vi "sample7(BlockR All).vi"() -> ()   [LabVIEW 2020]
uses:
  <vilib>/Platform/TimedLoop/XDataNode/timing_clust.ctl
  <vilib>/Platform/TimedLoop/XDataNode/nitl_modes.ctl
  <vilib>/Platform/TimedLoop/XDataNode/wakeup.ctl
  <vilib>/Platform/TimedLoop/XDataNode/XDataNode.xnode
  <vilib>/Platform/TimedLoop/XDataNode/XDNodeRunTimeDep.lvlib
panel:
  out "CtrlTable":u8[][](array[numeric]) format="%02x"
  out "波形チャート":u32(graph)
  out "cycle time":u32
  out "ModelName":string
  out "err":errorcluster caption="エラー出力" {"code" format="%04x"}
  out "present load":i16
  in  "UPDATE":bool
  out "ACK":bool
  in  "TorqueEnable":bool
  in  "OffsetTime":u32=500
  in  "frequency":dbl=0.2 min=0.0 max=10.0 step=0.05
  in  "waveform":enum16{"sin", "square"}(ring)
  in  "Target ID":u8=1 max=253
  in  "Baudrate":u32=1000000 min=9600 max=3000000 step=100
  in  "COM":refnum<visa-resource-name> caption="COMポート"
  in  "wave":bool
  out "Chart":T1(graph)
  out "STOP2":bool
  out "present position":i32
  in  "STOP":bool
  in  "goal position":i32(knob) scale=262144.0..-262144.0
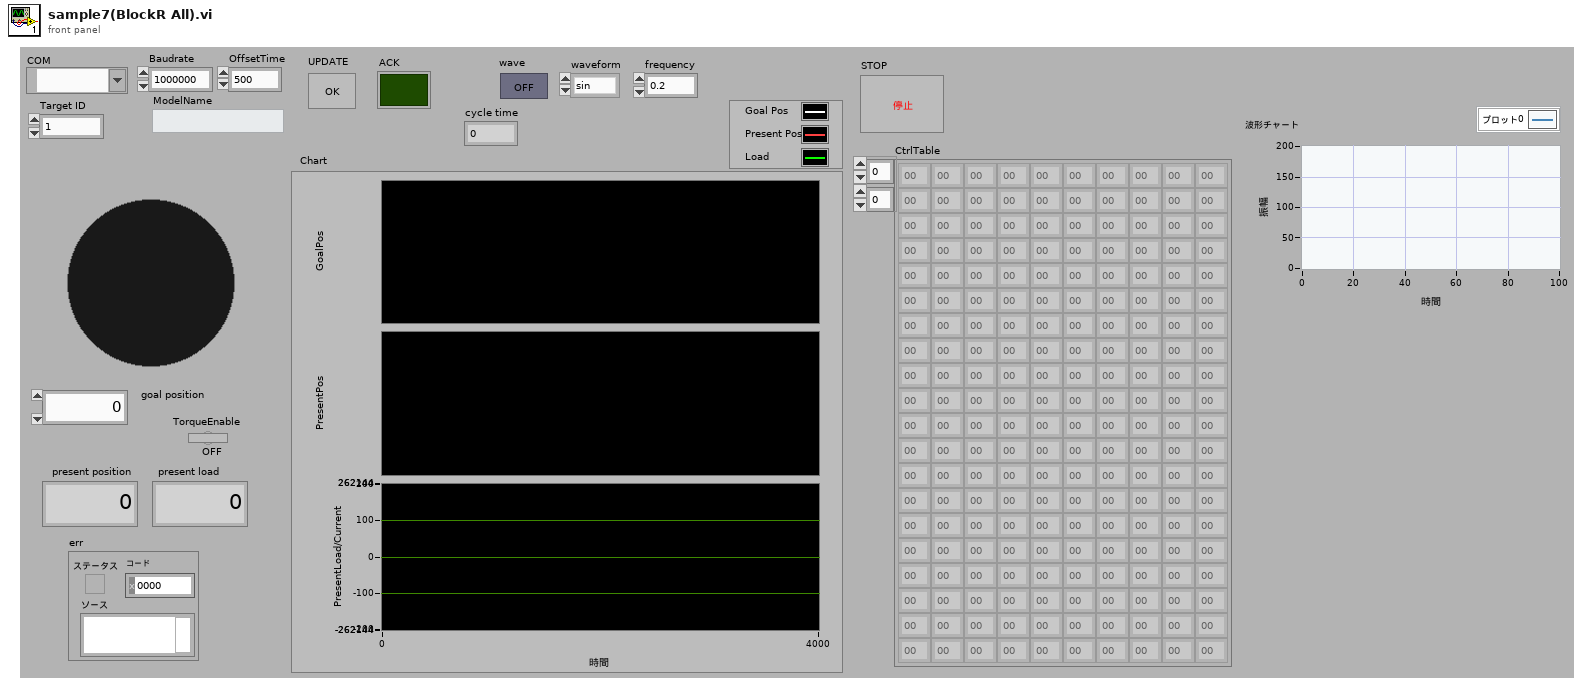
[diagram p1: front panel]
types:
  T1 = cluster{"goal position":i32, "present position":i32, "present load":i16}
  T2 = typedef "XDNodeRunTimeDep.lvlib/timing_clust.ctl" = cluster{"Expected End [f-1]":u64, "Actual End [f-1]":u64, "Finished Late? [f-1]":bool, "Expected End [i-1]":u64, "Actual End [i-1]":u64, "Finished Late? [i-1]":bool, "Expected Start [i]":u64, "Actual Start [i]":u64, "Expected Start [f]":u64, "Actual Start [f]":u64, "Source Name":string, "Structure Name":string, "Period":i64, "Deadline":i64, "Offset":i64, "Start":i64, "Priority":i32, "Timeout":i32, "Mode":T3, "Wakeup Reason":T4, "Error":errorcluster, "Source Type":string, "Secondary Source Type":string, "Global End Time":u64, "Global Start Time":u64, "Frame Duration":u64, "Iteration Duration":u64, "Assigned CPU":i32, "I/O Scan Engine Mode":u32}
  T3 = typedef "XDNodeRunTimeDep.lvlib/nitl_modes.ctl" = enum32{"No Change", "Process missed periods, maintain original phase", "Discard missed periods, maintain original phase", "Process missed periods, ignore original phase", "Discard missed periods, ignore original phase"}
  T4 = typedef "XDNodeRunTimeDep.lvlib/wakeup.ctl" = enum32{"Normal", "Aborted", "Asynchronous wakeup", "Timing source error", "Timed loop error", "Timeout"}
  T5 = cluster{"modelno":u16, "ModelName":string, "Type":enum8{"NONE", "DX", "AX", "RX", "EX", "MX", "XL320", "PRO", "PROP", "X", "Y"}, "MaxPosition":i32, "MinPosition":i32, "MaxAngle":dbl, "MinAngle":dbl, "MaxVelocity":i32, "MinVelocity":i32, "MaxPWM":i32, "MinPWM":i32, "VelocityRatio":dbl, "CurrentRatio":dbl, "PWMRatio":dbl}
  T6 = cluster{"ACK":bool, "ID":u8, "MaxPositionLimit":cluster{"address":u16, "width":u8, "limit":cluster{"max":i32, "min":i32}}, "MinPositionLimit":cluster{"address":u16, "width":u8, "limit":cluster{"max":i32, "min":i32}}, "TorqueEnable":cluster{"address":u16, "width":u8, "limit":cluster{"max":i32, "min":i32}}, "GoalPosition":cluster{"address":u16, "width":u8, "limit":cluster{"max":i32, "min":i32}}, "GoalVelocity":cluster{"address":u16, "width":u8, "limit":cluster{"max":i32, "min":i32}}, "PresentPosition":cluster{"address":u16, "width":u8, "limit":cluster{"max":i32, "min":i32}}, "PresentVelocity":cluster{"address":u16, "width":u8, "limit":cluster{"max":i32, "min":i32}}, "HardwareError":cluster{"address":u16, "width":u8, "limit":cluster{"max":i32, "min":i32}}}
  T7 = enum8{"NONE", "DX", "AX", "RX", "EX", "MX", "XL320", "PRO", "PROP", "X", "Y"}
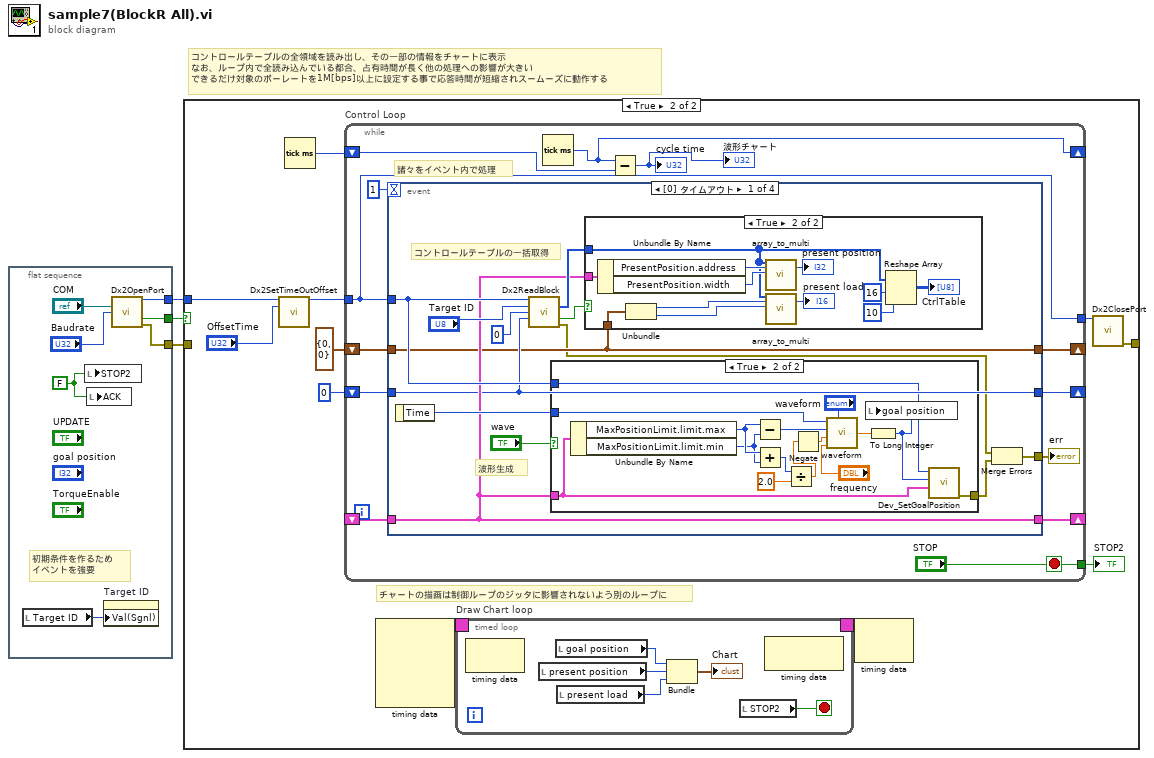
[diagram p0: block diagram]
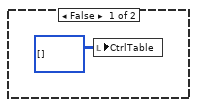
[diagram p4: hidden frame]
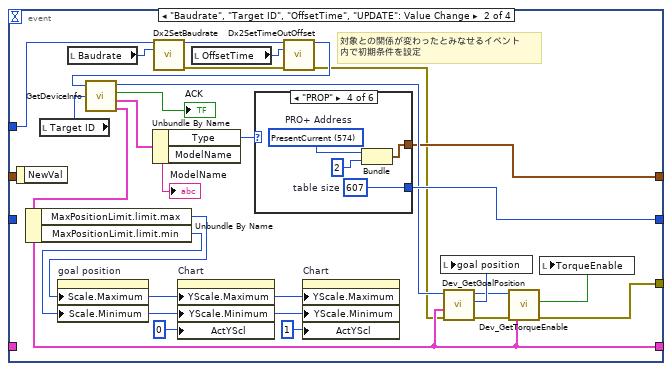
[diagram p5: hidden frame]
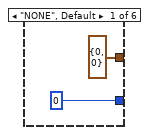
[diagram p6: hidden frame]
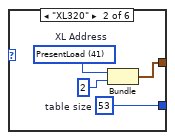
[diagram p7: hidden frame]
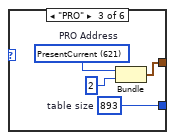
[diagram p8: hidden frame]
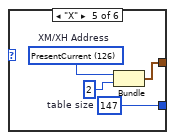
[diagram p9: hidden frame]
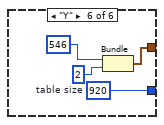
[diagram p10: hidden frame]
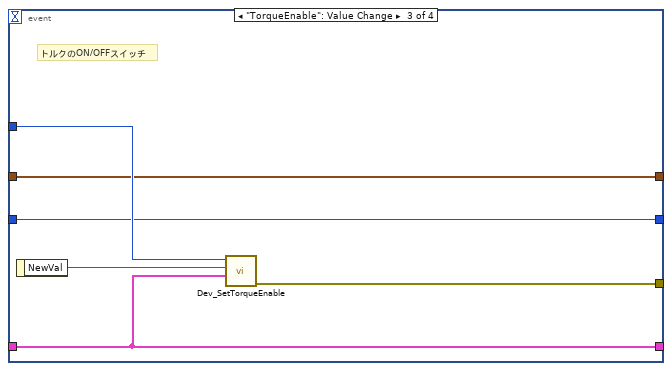
[diagram p11: hidden frame]
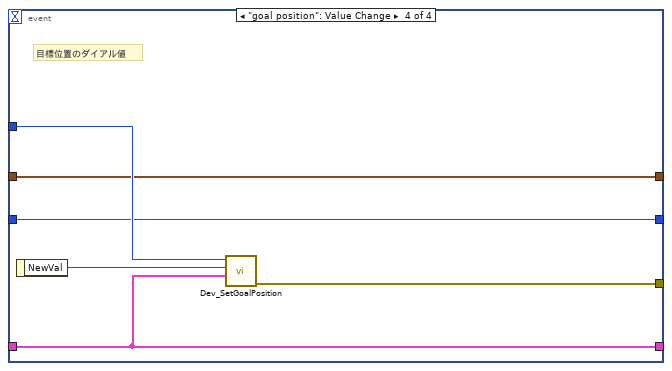
[diagram p12: hidden frame]
diagram:
  # "コントロールテーブルの全領域を読み出し、その一部の情報をチャートに表示\nなお、ループ内で全読み込んでいる都合、占有時間が長く他の処理への影響が大きい\nできるだけ対象のボーレートを1M[bps]以上に設定する事で応答時間が短縮されスームーズに動作する"
  n1 = flat-sequence {
    tunnel: [w10] -> w3
    tunnel: [w9] -> w2
    tunnel: [w8] -> w1
    frame #0 {
      w5 = FALSE ("停止 3")
      # "初期条件を作るため\nイベントを強要"
      n2 = local read "Target ID"() -> (w4:u8)
      n3 = local write "STOP2"(w5) -> ()
      n4 = local write "ACK"(w5) -> ()
      n5 = property on="Target ID" class="DigNum (指定)"("Val(Sgnl)"=w4) -> ()  [unwired: 2 in, 2 out]
      n6 = call "Dx2OpenPort.vi"("port"="COM", "baudrate"="Baudrate") -> ("dvid"=w9:u32, "成功"=w8:bool, "エラー出力"=w10:errorcluster)  [unwired: 11 in]
    }
  }
  n7 = case shown="TRUE" w1 {
    tunnel: w3 -> [w11 _]
    tunnel: w2 -> [_ w18]
    tunnel: [w11 w20] -> _
    frame False {
    }
    frame True {
      # "チャートの描画は制御ループのジッタに影響されないよう別のループに"
      n8 = call "Dx2SetTimeOutOffset.vi"("dvid in"=w18, "OffsetTime"="OffsetTime") -> ("dvid out"=w16:u32)  [unwired: 12 in, 1 out]
      n9 = Tick Count (ms)() -> (millisecond timer value=w12:u32)
      n10 = while "Control Loop" {
        shift-right: [w35] -> _
        shift-left: _ -> [w34]
        shift-right: [w33] -> _
        shift-left: u32 0 ("size") -> [w32]
        tunnel: w16 -> [w29]
        tunnel: ["STOP"] -> w17
        tunnel: [w29] -> w15
        shift-right: [w28] -> _
        shift-left: cluster{"XM/XM Address":u16, u8} {"XM/XM Address"=0, 0} -> [w27]
        shift-right: [w24] -> _
        shift-left: w12 -> [w25]
        stop <- "STOP" stop-if-true
        # "諸々をイベント内で処理"
        n11 = event shown="[0] タイムアウト" {
          selector: _ -> [_ _ _ _]
          dyn-events: _ -> [_ _ _ _]
          timeout: 1 -> [_ _ _ _]
          tunnel: [w41 w86 w127 w133] -> w35
          tunnel: w34 -> [w41 _ w127 w133]
          tunnel: [w38 w79 w124 w130] -> w26
          tunnel: [w40 w92 w126 w132] -> w33
          tunnel: w29 -> [w43 w91 w129 w134]
          tunnel: w32 -> [w40 _ w126 w132]
          tunnel: [w39 w87 w125 w131] -> w28
          tunnel: w27 -> [w39 _ w125 w131]
          event Timeout {
            # "波形生成"
            # "コントロールテーブルの一括取得"
            n12 = event-data() -> ("Time"=w44:u32)  [unwired: 1 in]
            n13 = call "Dx2ReadBlock.vi"("dvid in"=w43, "id"="Target ID", "address"=u16 0, "size"=w40) -> ("data out"=w47:u8[], "成功"=w46:bool, "エラー出力"=w36:errorcluster)  [unwired: 8 in, 1 out]
            n14 = case shown="TRUE" "wave" {
              tunnel: w41 -> [_ w51]
              tunnel: w44 -> [_ w63]
              tunnel: w43 -> [_ w61]
              tunnel: [_ w60] -> w37
              frame False {
              }
              frame True {
                n15 = Unbundle By Name(w51) -> ("MaxPositionLimit.limit.max"=w50:i32, "MaxPositionLimit.limit.min"=w49:i32)
                n16 = Subtract(x=w50, y=w49) -> (x-y=w57:i32)
                n17 = Add(x=w50, y=w49) -> (x+y=w56:i32)
                n18 = Divide(x=w56, y=2.0) -> (x/y=w55:dbl)
                n19 = Negate(x=w55) -> (-x=w52:dbl)
                n20 = call "waveform.vi"("time(ms)"=w63, "amplitude"=w57, "offset"=w52, "frequency"="frequency", "waveform"="waveform") -> ("wave"=w62:dbl)
                n21 = To Long Integer(number=w62) -> (32bit integer=w53:i32)
                n22 = local write "goal position"(w53) -> ()
                n23 = call "Dev_SetGoalPosition.vi"("ItemInfo"=w51, "goal position"=w53, "dvid in"=w61) -> ("エラー出力"=w60:errorcluster)  [unwired: 2 in, 2 out]
              }
            }
            n24 = case shown="TRUE" w46 {
              tunnel: w47 -> [_ w68]
              tunnel: w41 -> [_ w73]
              tunnel: w39 -> [_ w69]
              frame False {
                n25 = local write "CtrlTable"(u8[][] [] ("CtrlTable")) -> ()
              }
              frame True {
                n26 = Unbundle By Name(w73) -> ("PresentPosition.address"=w76:u16, "PresentPosition.width"=w75:u8)
                n27 = Unbundle(w69) -> ("XM/XM Address"=w71:u16, w70:u8)
                n28 = call "array_to_multi.vi"("array"=w68, "OffsetAddr"=w76, "length"=w75) -> ("uint32"=→"present position":u32)  [unwired: 16 in]
                n29 = call "array_to_multi.vi"("array"=w68, "OffsetAddr"=w71, "length"=w70) -> ("uint32"=→"present load":u32)  [unwired: 16 in]
                n30 = Reshape Array(w68, 16 ("次元サイズ"), 10 ("次元サイズ")) -> (→"CtrlTable":u8[][])
              }
            }
            n31 = Merge Errors(w36, w37) -> (w38:errorcluster)
          }
          event "Baudrate", "Target ID", "OffsetTime", "UPDATE": Value Change {
            # "対象との関係が変わったとみなせるイベント\n内で初期条件を設定"
            n32 = event-data() -> ()  [unwired: 1 in, 1 out]
            n33 = local read "Target ID"() -> (w95:u8)
            n34 = local read "Baudrate"() -> (w100:u32)
            n35 = call "Dx2SetBaudrate.vi"("dvid in"=w91, "Baudrate"=w100) -> ("dvid out"=w98:u32, "エラー出力"=w97:errorcluster)  [unwired: 11 in, 1 out]
            n36 = local read "OffsetTime"() -> (w99:u32)
            n37 = call "Dx2SetTimeOutOffset.vi"("dvid in"=w98, "OffsetTime"=w99, "エラー入力"=w97) -> ("dvid out"=w96:u32, "エラー出力"=w81:errorcluster)  [unwired: 11 in]
            n38 = call "GetDeviceInfo.vi"("dvid in"=w96, "Target ID"=w95) -> ("dvid out"=w90:u32, "matched"=→"ACK":bool, "ModelInfo"=w94:T5, "ItemInfo"=w86:T6)  [unwired: 1 in]
            n39 = Unbundle By Name(w86) -> ("MaxPositionLimit.limit.max"=w82:i32, "MaxPositionLimit.limit.min"=w83:i32)
            n40 = property on="goal position" class="Knob (指定)"("Scale.Maximum"=w82, "Scale.Minimum"=w83) -> ()  [unwired: 2 in, 2 out]
            n41 = Unbundle By Name(w94) -> ("Type"=w93:T7, "ModelName"=→"ModelName":string)
            n42 = property on="Chart" class="WFChart (指定)"("YScale.Maximum"=w82, "YScale.Minimum"=w83, "ActYScl"=0 ("アクティブYスケール")) -> ()  [unwired: 2 in, 2 out]
            n43 = case shown="\"PROP\"" w93 {
              tunnel: [u32 0 ("size") w107 w111 w115 w119 w123] -> w92
              tunnel: [cluster{"XM/XM Address":u16, u8} {"XM/XM Address"=0, 0} w104 w108 w113 w116 w121] -> w87
              frame "NONE", Default {
              }
              frame "XL320" {
                w106 = u16 41 items=["ModelNo"=0, "VersionOfFirmware"=2, "ID"=3, "Baudrate"=4, "ReturnDelayTime"=5, "CWAngleLimit"=6, "CCWAngleLimit"=8, "ControlMode"=11, "LimitTemperature"=12, "LowestLimitVoltage"=13, "HighestLimitVoltage"=14, "MaxTorque"=15, "StatusReturnLevel"=17, "AlarmShutdown"=18, "TorqueEnable"=24, "LED"=25, "DGain"=26, "IGain"=27, "PGain"=28, "GoalPosition"=30, "GoalVelocity"=32, "GoalTorque"=35, "PresentPosition"=37, "PresentSPeed"=39, "PresentLoad"=41, "PresentVoltage"=45, "PresentTemperature"=46, "RegistedInstruction"=47, "Moving"=49, "HardwareErrorStatus"=50, "Punch"=51]  # XL Address
                w107 = u32 53  # table size
                n44 = Bundle("XL Address"=w106, u8 2) -> (w104:cluster{"XL Address":u16, u8})  [unwired: 1 in]
              }
              frame "PRO" {
                w109 = u16 621 items=["ModelNo"=0, "ModelInfo"=2, "VersionOfFirmware"=6, "ID"=7, "Baudrate"=8, "ReturnDelayTime"=9, "OperationMode"=11, "HormingOffset"=13, "MovingThreshold"=17, "TemperatureLimit"=21, "MaxVoltageLimit"=22, "MinVoltageLimit"=24, "AccelerationLimit"=26, "TorqueLimit"=30, "VoltageLimit"=32, "MaxPositionLimit"=36, "MinPositionLimit"=40, "ExternalPortMode1"=44, "ExternalPortMode2"=45, "ExternalPortMode3"=46, "ExternalPortMode4"=47, "Shutdown"=48, "TorqueEnable"=562, "LED_Red"=563, "LED_Green"=564, "LED_Blue"=565, "VelocityIGain"=586, "VelocityPGain"=588, "PositionPGain"=594, "GoalPosition"=596, "GoalVelocity"=600, "GoalTorque"=604, "GoalAcceleration"=606, "Moving"=610, "PresentPosition"=611, "PresentVelocity"=615, "PresentCurrent"=621, "PresentInputVoltage"=623, "PresentTemperature"=625, "ExternalPortData1"=626, "ExternalPortData2"=628, "ExternalPortData3"=630, "ExternalPortData4"=632, "RegistedInstruction"=890, "StatusReturnLevel"=891, "HardwareError"=892]  # PRO Address
                w111 = u32 893  # table size
                n45 = Bundle("PRO Address"=w109, u8 2) -> (w108:cluster{"PRO Address":u16, u8})  [unwired: 1 in]
              }
              frame "PROP" {
                w112 = u16 574 items=["ModelNo"=0, "ModelInfo"=2, "VersionOfFirmware"=6, "ID"=7, "Baudrate"=8, "ReturnDelayTime"=9, "DriveMode"=10, "OperationMode"=11, "HormingOffset"=20, "MovingThreshold"=24, "TemperatureLimit"=31, "MaxVoltageLimit"=32, "MinVoltageLimit"=34, "PWMLimit"=36, "CurentLimit"=38, "AccelerationLimit"=40, "VelocitLimit"=44, "MaxPositionLimit"=48, "MinPositionLimit"=52, "ExternalPortMode1"=56, "ExternalPortMode2"=57, "ExternalPortMode3"=58, "ExternalPortMode4"=59, "Shutdown"=63, "TorqueEnable"=512, "LED_Red"=513, "LED_Green"=514, "LED_Blue"=515, "StatusReturnLevel"=516, "RegistedInstruction"=517, "HardwareErrorStatus"=518, "VelocityIGain"=524, "VelocityPGain"=526, "PositionDGain"=528, "PositionIGain"=530, "PositionPGain"=532, "PositionFF2ndGain"=536, "PositionFF1stGain"=538, "BusWatchdog"=546, "GoalPWM"=548, "GoalCurrent"=550, "GoalVelocity"=552, "ProfileAcceleration"=556, "ProfileVelocity"=560, "GoalPosition"=564, "RealtimeTick"=568, "Moving"=570, "MovingStatus"=571, "PresentPWM"=572, "PresentCurrent"=574, "PresentVelocity"=576, "PresentPosition"=580, "VelocityTrajectory"=584, "PositionTrajectory"=588, "PresentInputVoltage"=592, "PresentTemperature"=594, "ExternalPortData1"=600, "ExternalPortData2"=602, "ExternalPortData3"=604, "ExternalPortData4"=606]  # PRO+ Address
                w115 = u32 607  # table size
                n46 = Bundle("PRO+ Address"=w112, u8 2) -> (w113:cluster{"PRO+ Address":u16, u8})  [unwired: 1 in]
              }
              frame "X" {
                w117 = u16 126 items=["ModelNo"=0, "ModelInfo"=2, "VersionOfFirmware"=6, "ID"=7, "Baudrate"=8, "ReturnDelayTime"=9, "OperationMode"=11, "ProtocolVersion"=13, "HormingOffset"=20, "MovingThreshold"=24, "TemperatureLimit"=31, "MaxVoltageLimit"=32, "MinVoltageLimit"=34, "PWMLimit"=36, "CurrentLimit"=38, "AccelerationLimit"=40, "VelocityLimit"=44, "MaxPositionLimit"=48, "MinPositionLimit"=52, "Shutdown"=63, "TorqueEnable"=64, "LED"=65, "StatusReturnLevel"=68, "RegistedInstruction"=69, "HardwareErrorStatus"=70, "VelocityIGain"=76, "VelocityPGain"=78, "VelocityDGain"=80, "PositionIGain"=82, "PositionPGain"=84, "FeedForward2ndGain"=88, "FeedForward1stGain"=90, "GoalPWM"=100, "GoalCurrent"=102, "GoalVelocity"=104, "ProfileAcceleration"=108, "ProfileVelocity"=112, "GoalPosition"=116, "RealtimeTick"=120, "Moving"=122, "MovingStatus"=123, "PresentPWM"=124, "PresentCurrent"=126, "Presentvelocity"=128, "PresentPosition"=132, "VelocityTrajectory"=136, "PositionTrajectory"=140, "PresentIInputVoltage"=144, "PresentTemperature"=146]  # XM/XH Address
                w119 = u32 147  # table size
                n47 = Bundle("XM/XH Address"=w117, u8 2) -> (w116:cluster{"XM/XH Address":u16, u8})  [unwired: 1 in]
              }
              frame "Y" {
                w123 = u32 920  # table size
                n48 = Bundle(u16 546, u8 2) -> (w121:cluster{u16, u8})  [unwired: 1 in]
              }
            }
            n49 = property on="Chart" class="WFChart (指定)"("YScale.Maximum"=w82, "YScale.Minimum"=w83, "ActYScl"=1 ("アクティブYスケール")) -> ()  [unwired: 2 in, 2 out]
            n50 = call "Dev_GetGoalPosition.vi"("エラー入力"=w81, "ItemInfo"=w86, "dvid in"=w90) -> ("エラー出力"=w80:errorcluster, "goal position"=w89:i32, "dvid out"=w77:u32)  [unwired: 1 in, 1 out]
            n51 = local write "goal position"(w89) -> ()
            n52 = call "Dev_GetTorqueEnable.vi"("エラー入力"=w80, "ItemInfo"=w86, "dvid in"=w77) -> ("エラー出力"=w79:errorcluster, "torque enable"=w88:bool)  [unwired: 1 in, 2 out]
            n53 = local write "TorqueEnable"(w88) -> ()
          }
          event "TorqueEnable": Value Change {
            # "トルクのON/OFFスイッチ"
            n54 = event-data() -> ("NewVal"=w128:bool)  [unwired: 1 in]
            n55 = call "Dev_SetTorqueEnable.vi"("ItemInfo"=w127, "torque enable"=w128, "dvid in"=w129) -> ("エラー出力"=w124:errorcluster)  [unwired: 2 in, 2 out]
          }
          event "goal position": Value Change {
            # "目標位置のダイアル値"
            n56 = event-data() -> ("NewVal"=w135:i32)  [unwired: 1 in]
            n57 = call "Dev_SetGoalPosition.vi"("ItemInfo"=w133, "goal position"=w135, "dvid in"=w134) -> ("エラー出力"=w130:errorcluster)  [unwired: 2 in, 2 out]
          }
        }
        "err" <- w26
        n58 = Tick Count (ms)() -> (millisecond timer value=w24:u32)
        n59 = Subtract(x=w24, y=w25) -> (x-y=→"cycle time" →"波形チャート":u32)
      }
      "STOP2" <- w17
      n60 = node-c288() -> (w22:T2)  [unwired: 4 in]
      n61 = timed-loop "Draw Chart loop" {
        timing: w22 -> [_]
        timing-out: [_] -> w21
        stop <- w140 stop-if-true
        n62 = node-c288() -> ()  [unwired: 1 in, 1 out]
        n63 = local read "present position"() -> (w138:i32)
        n64 = local read "goal position"() -> (w139:i32)
        n65 = local read "present load"() -> (w136:i16)
        n66 = Bundle("goal position"=w139, "present position"=w138, "present load"=w136) -> (→"Chart":T1)  [unwired: 1 in]
        n67 = local read "STOP2"() -> (w140:bool)
        n68 = node-c288() -> ()  [unwired: 1 in, 1 out]
      }
      n69 = node-c288(w21) -> ()  [unwired: 1 out]
      n70 = call "Dx2ClosePort.vi"("dvid"=w15) -> ("エラー出力"=w20:errorcluster)  [unwired: 13 in, 1 out]
    }
  }
